vi "Global Shutter Variables - SubVI.vi"() -> ()   [LabVIEW 2014]
panel:
  in  "Laser Shutter":T1(radio)
  in  "Camera Shutter 2":bool
  in  "Wheel Speed":u8=1 min=1 max=7 step=1
  out "Camera Shutter":bool[](array[boolean])
  out "Shutter In Use":string
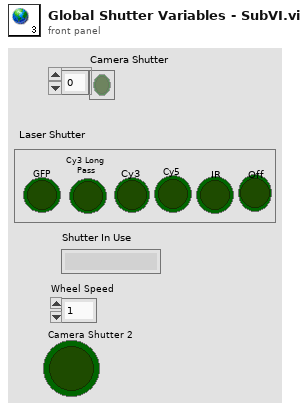
[diagram p1: front panel]
types:
  T1 = enum32{"No Selection", "GFP", "Cy3 Long \nPass", "Cy3", "Cy5", "Off", "IR"}
diagram:
